vi "CheckRTTargetModel.vi"(8 "error in (no error)":errorcluster, 10 "Supported Devices":u32[](array[numeric]), 11 "IP or Hostname":string) -> (0 "error out":errorcluster, 3 "RT Target Info":T1)   [LabVIEW 2021, in "myRIOMetaDataObj.lvclass"]
uses:
  myRIOMetaDataObj.lvclass
  <vilib>/nisyscfg/Close (System).vi
  <resource>/objmgr/nisysapi.rc
  <resource>/myRIO/Target Info.ctl
  <vilib>/Utility/error.llb/DialogType.ctl
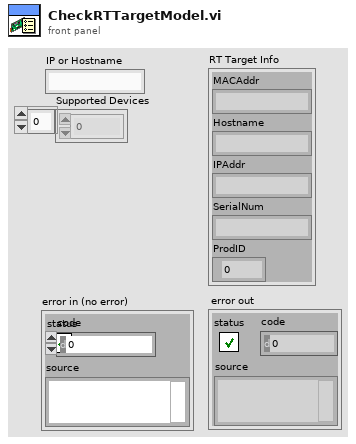
[diagram p1: front panel]
types:
  T1 = typedef "Target Info.ctl" = cluster{"MACAddr":string, "Hostname":string, "IPAddr":string, "SerialNum":string, "ProdID":u32}
  T2 = typedef "DialogType.ctl" = u16
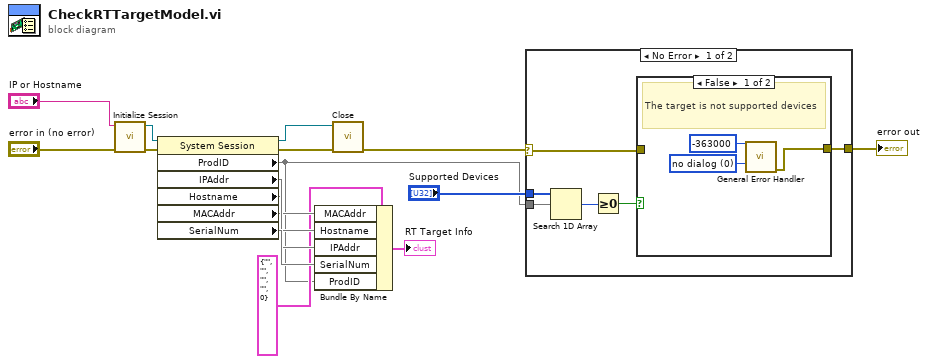
[diagram p0: block diagram]
diagram:
  n1 = call <vilib>:"Initialize Session.vi"("error in (no error)"="error in (no error)", "Target (localhost)"="IP or Hostname") -> ("error out"=w8:errorcluster, "Session out"=w7:refnum<k21>)  [unwired: 8 in]
  n2 = property class="System Session"(reference=w7, error in=w8) -> (reference out=w10:refnum<k21>, error out=w9:errorcluster, "ProdID"=w3, "IPAddr"=w14, "Hostname"=w13, "MACAddr"=w12, "SerialNum"=w15)
  n3 = Bundle By Name(cluster=T1 {"MACAddr"="", "Hostname"="", "IPAddr"="", "SerialNum"="", "ProdID"=0} ("Target Info"), "MACAddr"=w12, "Hostname"=w13, "IPAddr"=w14, "SerialNum"=w15, "ProdID"=w3) -> (→"RT Target Info":T1)
  n4 = call-poly <vilib>:"Close.vi"("error in (no error)"=w9, "Session in"=w10) -> ("error out"=w2:errorcluster)  [unwired: 9 in]
  n5 = case shown="No Error" w2 {
    selector: w2 -> [w21 w27]
    tunnel: "Supported Devices" -> [w20 _]
    tunnel: w3 -> [w19 _]
    tunnel: [w22 w27] -> w1
    frame No Error {
      n6 = Search 1D Array(1D array=w20, element=w19) -> (index of element=w18:i32)  [unwired: 1 in]
      n7 = Greater Or Equal To 0?(x=w18) -> (x >= 0?=w17:bool)
      n8 = case shown="False" w17 {
        tunnel: w21 -> [_ w26]
        tunnel: [w24 w26] -> w22
        frame False {
          w25 = T2 0 items=["no dialog", "OK message", "continue or stop message", "OK message + warnings", "continue/stop + warnings"] ("type of dialog (OK msg:1)")
          # "The target is not supported devices"
          n9 = call <vilib>:"General Error Handler.vi"("[error code] (0)"=-363000, "type of dialog (OK msg:1)"=w25) -> ("error out"=w24:errorcluster)  [unwired: 9 in, 4 out]
        }
        frame True {
          # "The target is supported devices"
        }
      }
    }
    frame Error {
    }
  }
  "error out" <- w1
